vi "SD-Write Key (Path).vi"(7 "section":string, 8 "error in (no error)":errorcluster, 9 "value":path, 10 "key":string, 11 "refnum":T1) -> (0 "error out":errorcluster, 2 "found?":bool, 3 "refnum out":T1)   [LabVIEW 2020, in "SD-NI_LVConfig.lvlib"]
doc: "Writes a value to a key in a specified section of the configuration data identified by <B>refnum</B>. This VI modifies data in memory. To write data to disk, use the Close Config Data VI. Wire data to the <B>value</B> input to determine the polymorphic instance to use or manually select the instance."
uses:
  SD-NI_LVConfig.lvlib
  SD-Config Data RefNum.ctl
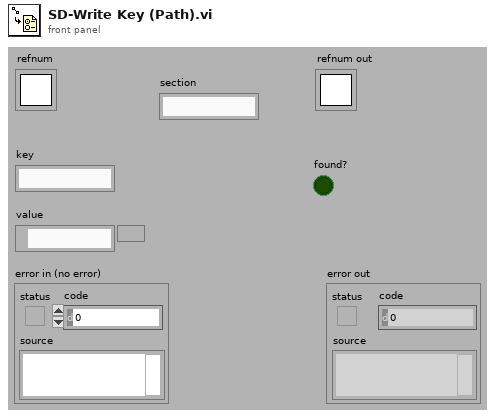
[diagram p1: front panel]
types:
  T1 = typedef "SD-NI_LVConfig.lvlib/SD-Config Data RefNum.ctl" = refnum<k1>
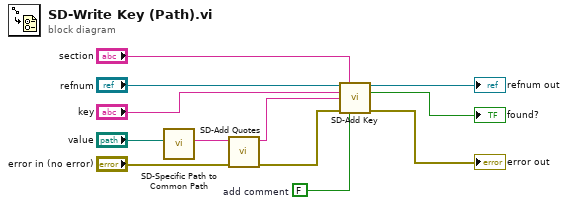
[diagram p0: block diagram]
diagram:
  w5 = FALSE  # add comment
  n1 = call "SD-Specific Path to Common Path.vi"("specific path"="value") -> ("common path"=w4:string)  [unwired: 10 in]
  n2 = call "SD-Add Quotes.vi"("error in (no error)"="error in (no error)", "string"=w4) -> ("error out"=w1:errorcluster, "with quotes"=w2:string)  [unwired: 8 in]
  n3 = call "SD-Add Key.vi"("refnum"="refnum", "section"="section", "key"="key", "value"=w2, "error in (no error)"=w1, "add comment"=w5) -> ("refnum out"=→"refnum out":T1, "key exists?"=→"found?":bool, "error out"=→"error out":errorcluster)  [unwired: 7 out]
